vi "Lookup Entity Enqueuer.vi"(8 "error in (no error)":errorcluster, 9 "entity type":i32, 10 "entity index":i32, 11 "entity table in":refnum<class "Entity Table.lvclass">) -> (0 "error out":errorcluster, 2 "entity":refnum<class "Message Enqueuer.lvclass">, 3 "entity table out":refnum<class "Entity Table.lvclass">)   [LabVIEW 2023, in "Entity Table.lvclass"]
doc: "Look up the enqueuer of an Actor contained in the entity table by index and type."
uses:
  Entity Table.lvclass
  <vilib>/ActorFramework/Message Enqueuer/Message Enqueuer.lvclass
  Entity Table.lvclass/Entity Table.ctl
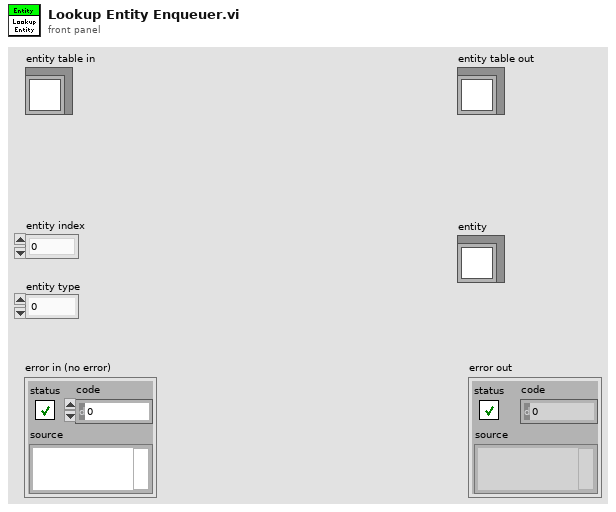
[diagram p1: front panel]
types:
  T1 = typedef "Entity Table.lvclass/Entity Table Element.ctl" = cluster{"Entity":refnum<class "Message Enqueuer.lvclass">[], "Entity Data":T2[]}
  T2 = typedef "Entity Table.lvclass/Entity Data.ctl" = cluster{"Name":string, "Status":string}
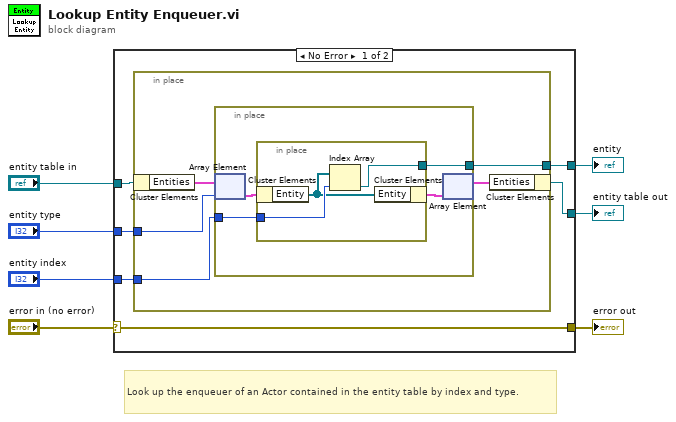
[diagram p0: block diagram]
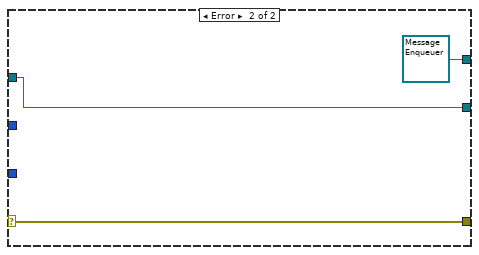
[diagram p2: hidden frame]
diagram:
  # "Look up the enqueuer of an Actor contained in the entity table by index and type."
  n1 = case shown="No Error" "error in (no error)" {
    selector: "error in (no error)" -> [w10 w28]
    tunnel: [w10 w28] -> w6
    tunnel: "entity table in" -> [w9 w27]
    tunnel: [w8 w27] -> w4
    tunnel: [w11 refnum<class "Message Enqueuer.lvclass"> refnum ("entity")] -> w3
    tunnel: "entity type" -> [w13 _]
    tunnel: "entity index" -> [w12 _]
    frame No Error {
      n2 = in-place "In Place Element Structure" {
        in-place-border: w13 -> [w18]
        in-place-border: w12 -> [w17]
        in-place-border: [w16] -> w11
        n3 = in-place-cluster #1 ("Unbundle / Bundle Elements")(w9) -> ("Entities"=w15:T1[])
        n4 = in-place "In Place Element Structure" {
          in-place-border: w17 -> [w21]
          in-place-border: [w20] -> w16
          n5 = in-place-array #2 ("Array Index / Replace Elements")(w15, w18) -> (w22:T1)
          n6 = in-place "In Place Element Structure" {
            in-place-border: w21 -> [w25]
            in-place-border: [w23] -> w20
            n7 = in-place-cluster #3 ("Unbundle / Bundle Elements")(w22) -> ("Entity"=w24:refnum<class "Message Enqueuer.lvclass">[])
            n8 = Index Array(array=w24, index=w25) -> (element=w23:refnum<class "Message Enqueuer.lvclass">)
            n9 = in-place-cluster #3 ("Unbundle / Bundle Elements")("Entity"=w24) -> (w19:T1)
          }
          n10 = in-place-array #2 ("Array Index / Replace Elements")(w19) -> (w14:T1[])  [unwired: 1 out]
        }
        n11 = in-place-cluster #1 ("Unbundle / Bundle Elements")("Entities"=w14) -> (w8:refnum<class "Entity Table.lvclass">)
      }
    }
    frame Error {
    }
  }
  "error out" <- w6
  "entity" <- w3
  "entity table out" <- w4
